vi "Pack for gRPC.vi"(8 "error in":errorcluster, 9 "configuration / results":enum16{"Configuration", "Results"}(ring), 10 "data value":variant, 11 "measurement customizations in":refnum<class "Measurement Plugin.lvclass">) -> (0 "error out":errorcluster, 2 "any":T1, 3 "measurement customizations out":refnum<class "Measurement Plugin.lvclass">)   [LabVIEW 2021, in "Load Transient Response with Pin Map.lvlib" / "Measurement Plugin.lvclass"]
uses:
  Measurement Plugin.lvclass
  Measurement Configuration.ctl
  Load Transient Response with Pin Map.lvlib
  Measurement Results.ctl
  a6012965-5700-4384-8228-972e71b6560c.vi
  2eca732d-dbaa-43bf-a7dd-ede2da65bc1b.vi
  <vilib>/Plug-In SDKs/Measurements/Measurement Plugin Service/Measurement Plugin Service.lvclass
  <instrlib>/niScope/Controls/niScope vertical coupling.ctl
  <vilib>/gRPC/LabVIEW gRPC Library/Shared/Any.ctl
  <vilib>/gRPC/LabVIEW gRPC Library/grpc-lvsupport-release.lvlib
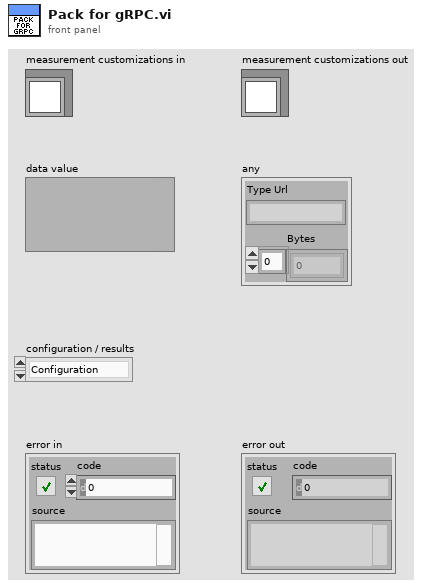
[diagram p1: front panel]
types:
  T1 = typedef "grpc-lvsupport-release.lvlib/Any.ctl" = cluster{"Type Url":string, "Bytes":u8[]}
  T2 = typedef "grpc-lvsupport-release.lvlib/grpcId.ctl" = u64
  T3 = typedef "Load Transient Response with Pin Map.lvlib/Measurement Configuration.ctl" = cluster{"Mode of operation":enum32{"Power on the DUT", "Perform measurement", "Power off the DUT"}, "DUT setup time":dbl, "Nominal output voltage":dbl, "Source pin name":string, "Source sense":i32, "Source current limit":dbl, "Source voltage level":dbl, "Source transient response":i32, "Source voltage gain bandwidth":dbl, "Source voltage compensation frequency":dbl, "Source voltage pole-zero ratio":dbl, "Load pin name":string, "Load sense":i32, "Load voltage limit range":dbl, "Load current level range":dbl, "Load sample rate":dbl, "Load current set point 1":dbl, "Load current set point 2":dbl, "Load current delay t1":dbl, "Load current pulse duration":dbl, "Load current delay t2":dbl, "Load current rising slew rate":dbl, "Load current falling slew rate":dbl, "Load transient response":i32, "Load current gain bandwidth":dbl, "Load current compensation frequency":dbl, "Load current pole-zero ratio":dbl, "Pin Names for Scope":string[], "vertical range":dbl[], "vertical offset":dbl[], "probe attenuation":dbl[], "vertical coupling":T4[], "input impedance":u32[], "max input frequency":dbl[], "min record length":i32[], "channel enabled":bool[], "enforce realtime":bool[], "reference position":dbl[], "min sample rate":dbl[]}
  T4 = typedef "niScope vertical coupling.ctl" = i32
  T5 = typedef "Load Transient Response with Pin Map.lvlib/Measurement Results.ctl" = cluster{"Status":string, "dt":dbl, "Load voltages":dbl[], "Load currents":dbl[], "Undershoot load voltage":dbl, "Overshoot load voltage":dbl, "waveform pins":string[], "waveform sites":i32[], "waveform t0 array":dbl[], "waveform dt array":dbl[], "waveform length array":i32[], "concatenated waveform Y":dbl[]}
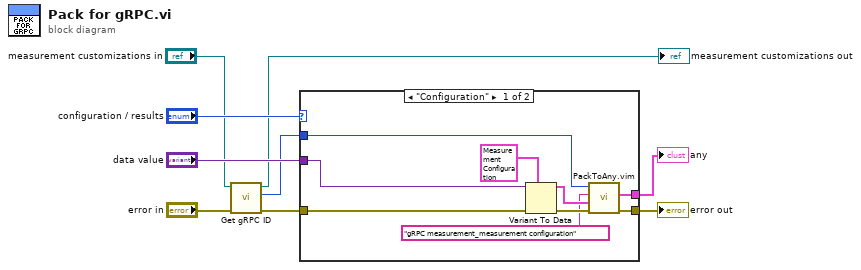
[diagram p0: block diagram]
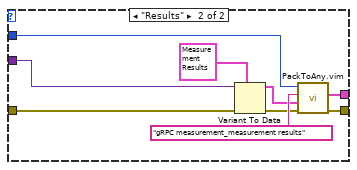
[diagram p2: hidden frame]
diagram:
  n1 = call <vilib>:"Get gRPC ID.vi"("error in"="error in", "measurement plugin service in"="measurement customizations in") -> ("error out"=w4:errorcluster, "gRPC ID"=w1:T2, "measurement plugin service out"=→"measurement customizations out":refnum<class "Measurement Plugin.lvclass">)  [unwired: 7 in]
  n2 = case shown="\"Configuration\"" "configuration / results" {
    tunnel: w4 -> [w18 w27]
    tunnel: "data value" -> [w17 w26]
    tunnel: w1 -> [w14 w22]
    tunnel: [w16 w24] -> w8
    tunnel: [w15 w23] -> w7
    frame "Configuration" {
      n3 = Variant To Data(error in=w18, type=T3 {"Mode of operation"=enum."Perform measurement", "DUT setup time"=1.2, "Nominal output voltage"=32.0, "Source pin name"="Lorem ipsum dolor sit", "Source sense"=64, "Source current limit"=64.0, "Source voltage level"=-32.0, "Source transient response"=-32, "Source voltage gain bandwidth"=-64.0, "Source voltage compensation frequency"=-64.0, "Source voltage pole-zero ratio"=1.0, "Load pin name"="Lorem ipsum dolor sit", "Load sense"=1, "Load voltage limit range"=1.0, "Load current level range"=40.0, "Load sample rate"=1800000.0, "Load current set point 1"=4.0, "Load current set point 2"=14.0, "Load current delay t1"=0.001, "Load current pulse duration"=0.001, "Load current delay t2"=0.001, "Load current rising slew rate"=24.0, "Load current falling slew rate"=24.0, "Load transient response"=1042, "Load current gain bandwidth"=14000.0, "Load current compensation frequency"=180000.0, "Load current pole-zero ratio"=0.3, "Pin Names for Scope"=[], "vertical range"=[], "vertical offset"=[], "probe attenuation"=[], "vertical coupling"=[], "input impedance"=[], "max input frequency"=[], "min record length"=[], "channel enabled"=[], "enforce realtime"=[], "reference position"=[], "min sample rate"=[]} ("measurement configuration"), Variant=w17) -> (data=w13:T3, error out=w12:errorcluster)
      n4 = call "PackToAny.vim"("error in"=w12, "Data To Pack"=w13, "Message Type"="gRPC measurement_measurement configuration", "gRPCid in"=w14) -> ("error out"=w16:errorcluster, "Any"=w15:T1)  [unwired: 5 in, 1 out]
    }
    frame "Results" {
      n5 = Variant To Data(error in=w27, type=T5 {"Status"="Empty", "dt"=0.0, "Load voltages"=[], "Load currents"=[], "Undershoot load voltage"=0.0, "Overshoot load voltage"=0.0, "waveform pins"=[], "waveform sites"=[], "waveform t0 array"=[], "waveform dt array"=[], "waveform length array"=[], "concatenated waveform Y"=[]} ("Measurement Results"), Variant=w26) -> (data=w20:T5, error out=w19:errorcluster)
      n6 = call "PackToAny.vim"("error in"=w19, "Data To Pack"=w20, "Message Type"="gRPC measurement_measurement results", "gRPCid in"=w22) -> ("error out"=w24:errorcluster, "Any"=w23:T1)  [unwired: 5 in, 1 out]
    }
  }
  "error out" <- w8
  "any" <- w7
